vi "Example_SVM.vi"() -> ()   [LabVIEW 2009]
uses:
  <vilib>/Utility/miscctls.llb/LV3DPointTypeDef.ctl
  <vilib>/addons/Machine Learning/Visualization/Visualization (3D).vi
  <vilib>/gmath/interp.llb/Create Mesh Grid (2D) (x,y arrays).vi
  <vilib>/addons/Machine Learning/NILabs_MLT.lvlib
  <vilib>/gmath/NI_Gmath.lvlib
  <vilib>/Analysis/NI_AALBase.lvlib
panel:
  in  "# of samples":i32=200
  in  "Soft margin parameter":dbl=2.0
  in  "Parameter":dbl=2.0
  in  "Kernel type":T1(ring)=enum."Gaussian Kernel"
  out "Test Data":refnum<vi>(3d-picture)
  out "Training Data":refnum<vi>(3d-picture)
  # "Introduction:\nSupport Vector Machine (SVM) is applied to a classification problem, where the training set contains two concentric circles. The learned SVM is used to classify data drawn from a unform distribution, so that the classification boundary can be seen."
  # "(Samples are overlain with predicted class labels.)"
  # "(Samples are overlain with class labels.)"
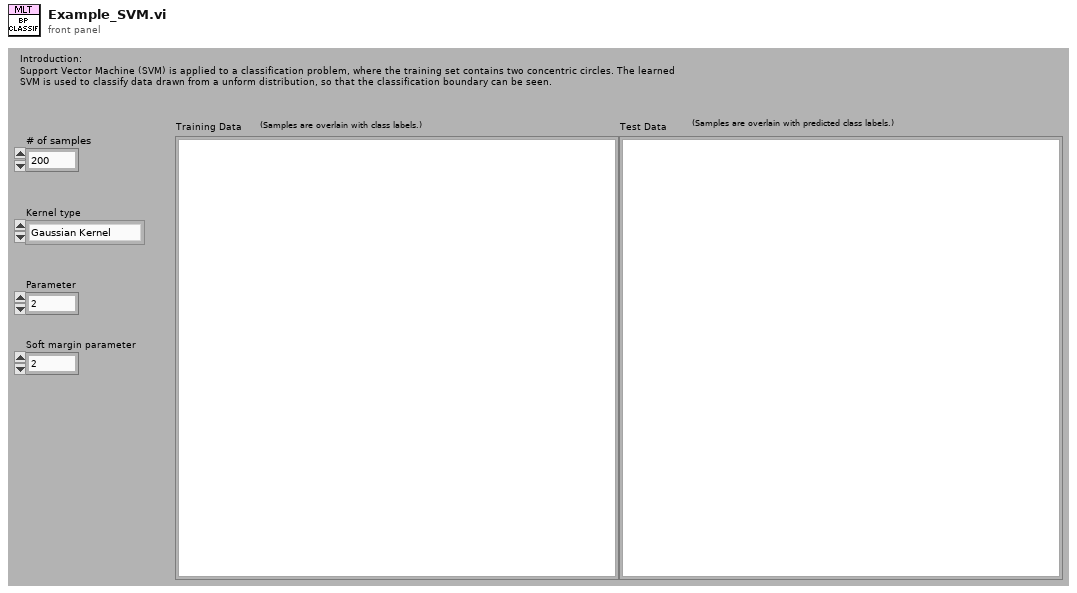
[diagram p1: front panel]
types:
  T1 = enum16{"Linear Kernel", "Polynomial Kernel", "Gaussian Kernel"}
  T2 = typedef "LV3DPointTypeDef.ctl" = cluster{"X":sgl, "Y":sgl, "Z":sgl}
  T3 = typedef "NILabs_MLT.lvlib/ml_SVM_Project.ctl" = cluster{"X":variant[], "y":dbl[], "Kernel Function":refnum<vi>, "parameters":variant, "soft margin parameter":dbl, "alpha":dbl[], "b":dbl}
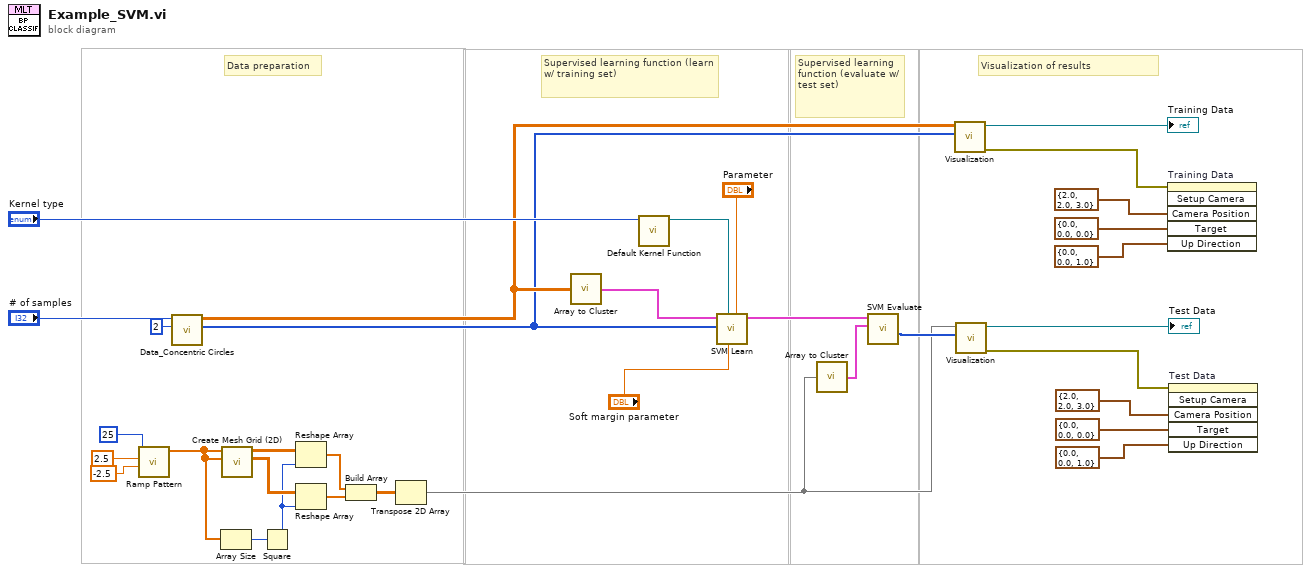
[diagram p0: block diagram]
diagram:
  # "Visualization of results"
  # "Supervised learning function (evaluate w/ test set)"
  # "Supervised learning function (learn w/ training set)"
  # "Data preparation"
  n1 = call <vilib>:"Ramp Pattern.vi"("start"=-2.5, "end"=2.5, "samples"=25) -> ("Ramp Pattern"=w11:dbl[])  [unwired: 7 in, 1 out]
  n2 = call "Data_Concentric Circles.vi"("# of circles"=2, "# of points"="# of samples") -> ("Classes"=w1:i32[], "Data"=w2:dbl[][])  [unwired: 8 in]
  n3 = Array Size(array=w11) -> (size(s)=w10:i32)
  n4 = call-poly <vilib>:"Create Mesh Grid (2D).vi"("y domain"=w11, "x domain"=w11) -> ("Y"=w12:dbl[][], "X"=w13:dbl[][])  [unwired: 7 in, 1 out]
  n5 = Square(x=w10) -> (x^2=w9:i32)
  n6 = Reshape Array(w13, w9) -> (w8:dbl[])
  n7 = Reshape Array(w12, w9) -> (w7:dbl[])
  n8 = Build Array(w8, w7) -> (w6:dbl[][])
  n9 = Transpose 2D Array(2D array=w6) -> (transposed array=w5:dbl[][])
  n10 = call <vilib>:"Array to Cluster.vi"("Data in Array"=w2) -> ("Data in Cluster"=w23:cluster{"Sample":dbl[]}[])
  n11 = call <vilib>:"Default Kernel Function.vi"("kernel type"="Kernel type") -> ("Kernel Function"=w22:refnum<vi>)  [unwired: 9 in, 1 out]
  n12 = call <vilib>:"SVM Learn.vi"("parameters"="Parameter", "soft margin parameter"="Soft margin parameter", "Kernel Function"=w22, "Class labels"=w1, "Data samples"=w23) -> ("SVM"=w19:T3)  [unwired: 5 in, 1 out]
  n13 = call <vilib>:"Array to Cluster.vi"("Data in Array"=w5) -> ("Data in Cluster"=w20:cluster{"Sample":dbl[]}[])
  n14 = call <vilib>:"SVM Evaluate.vi"("Data samples"=w20, "SVM"=w19) -> ("Class labels"=w18:i32[])  [unwired: 6 in, 3 out]
  n15 = call-poly <vilib>:"Visualization.vi"("Class labels"=w1, "Data samples"=w2) -> ("error out"=w29:errorcluster, "3D Picture"=→"Training Data":refnum<vi>)  [unwired: 8 in]
  n16 = call-poly <vilib>:"Visualization.vi"("Class labels"=w18, "Data samples"=w5) -> ("error out"=w28:errorcluster, "3D Picture"=→"Test Data":refnum<vi>)  [unwired: 8 in]
  n17 = invoke on="Training Data" class="SceneGraphDisp (strict)" method="Setup Camera"(error in=w29, "Camera Position"=T2 {"X"=2.0, "Y"=2.0, "Z"=3.0}, "Target"=T2 {"X"=0.0, "Y"=0.0, "Z"=0.0} ("Camera Position"), "Up Direction"=T2 {"X"=0.0, "Y"=0.0, "Z"=1.0} ("Camera Position")) -> ()  [unwired: 2 in, 6 out]
  n18 = invoke on="Test Data" class="SceneGraphDisp (strict)" method="Setup Camera"(error in=w28, "Camera Position"=T2 {"X"=2.0, "Y"=2.0, "Z"=3.0}, "Target"=T2 {"X"=0.0, "Y"=0.0, "Z"=0.0} ("Camera Position"), "Up Direction"=T2 {"X"=0.0, "Y"=0.0, "Z"=1.0} ("Camera Position")) -> ()  [unwired: 2 in, 6 out]
